vi "saveTimeSeries_III.vi"(0 "422nm":dbl, 1 "file path (dialog if empty)":path, 2 "save?":bool, 5 "532nm":dbl, 7 "785nm":dbl, 11 "Error In":errorcluster) -> (15 "Error Out":errorcluster)   [LabVIEW 2011]
uses:
  <vilib>/Utility/file.llb/Write To Spreadsheet File (string).vi
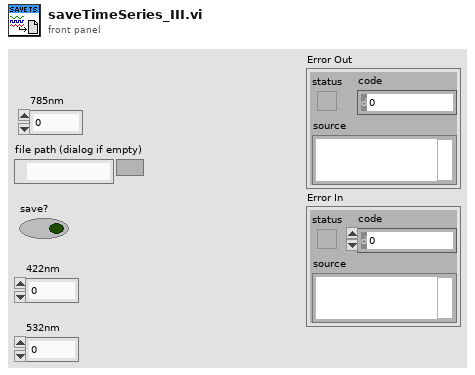
[diagram p1: front panel]
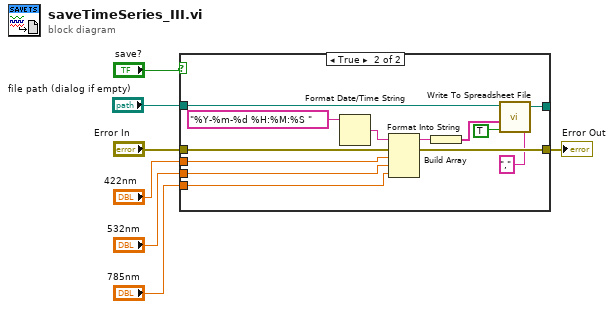
[diagram p0: block diagram]
diagram:
  n1 = case shown="True" "save?" {
    tunnel: "785nm" -> [_ w22]
    tunnel: "532nm" -> [_ w21]
    tunnel: "422nm" -> [_ w20]
    tunnel: "file path (dialog if empty)" -> [w9 w19]
    tunnel: [w9 w18] -> _
    tunnel: "Error In" -> [w8 w12]
    tunnel: [w8 w11] -> w3
    frame False {
    }
    frame True {
      n2 = Format Date/Time String(time format string (%c)="%Y-%m-%d %H:%M:%S ") -> (date/time string=w16:string)  [unwired: 2 in]
      n3 = Format Into String(initial string=w16, error in=w12, w20, w21, w22) -> (resulting string=w14:string, error out=w11:errorcluster)  [unwired: 1 in]
      n4 = Build Array(w14) -> (w13:string[])
      n5 = call-poly <vilib>:"Write To Spreadsheet File.vi"("delimiter (\\t)"="," ("delimiter (\\t)"), "append to file? (new file:F)"=TRUE, "1D data"=w13, "file path (dialog if empty)"=w19) -> ("new file path (Not A Path if cancelled)"=w18:path)  [unwired: 4 in]
    }
  }
  "Error Out" <- w3
